vi "Analysis.Result Summaries, Generate Yield Per Day.vi"(9 "Type":enum16{"First Pass", "Last Pass", "All"}(ring), 11 "ResultSum":T1[](array[typedef])) -> (2 "Yield Per Date":string[][](table), 3 "Yield vs Date":cluster{timestamp[], dbl[]}(graph))   [LabVIEW 2024]
uses:
  Analysis.Result Summary.ctl
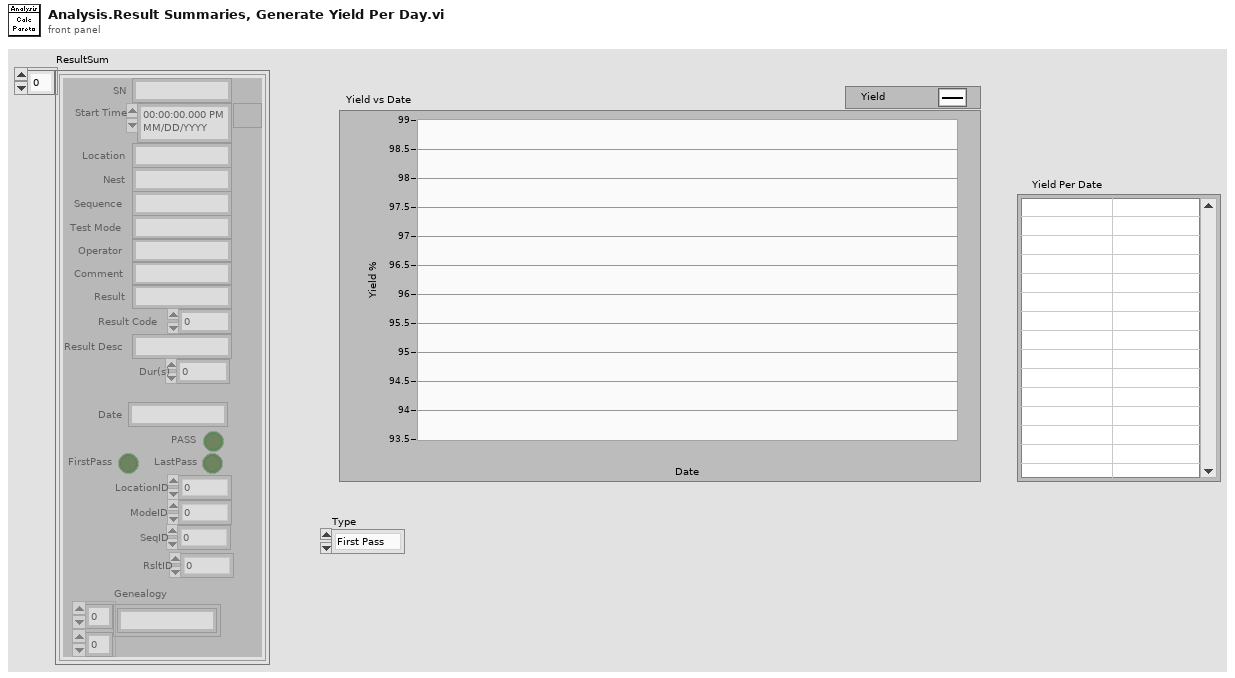
[diagram p1: front panel]
types:
  T1 = typedef "Analysis.Result Summary.ctl" = cluster{"SN":string, "Start Time":timestamp, "Location":string, "Nest":string, "Sequence":string, "Operator":string, "Test Mode":string, "Comment":string, "Result":string, "Result Code":i32, "Result Desc":string, "Date":string, "Dur(s)":dbl, "PASS":bool, "FirstPass":bool, "LastPass":bool, "LocationID":i32, "ModeID":i32, "SeqID":i32, "RsltID":i32, "Genealogy":string[][]}
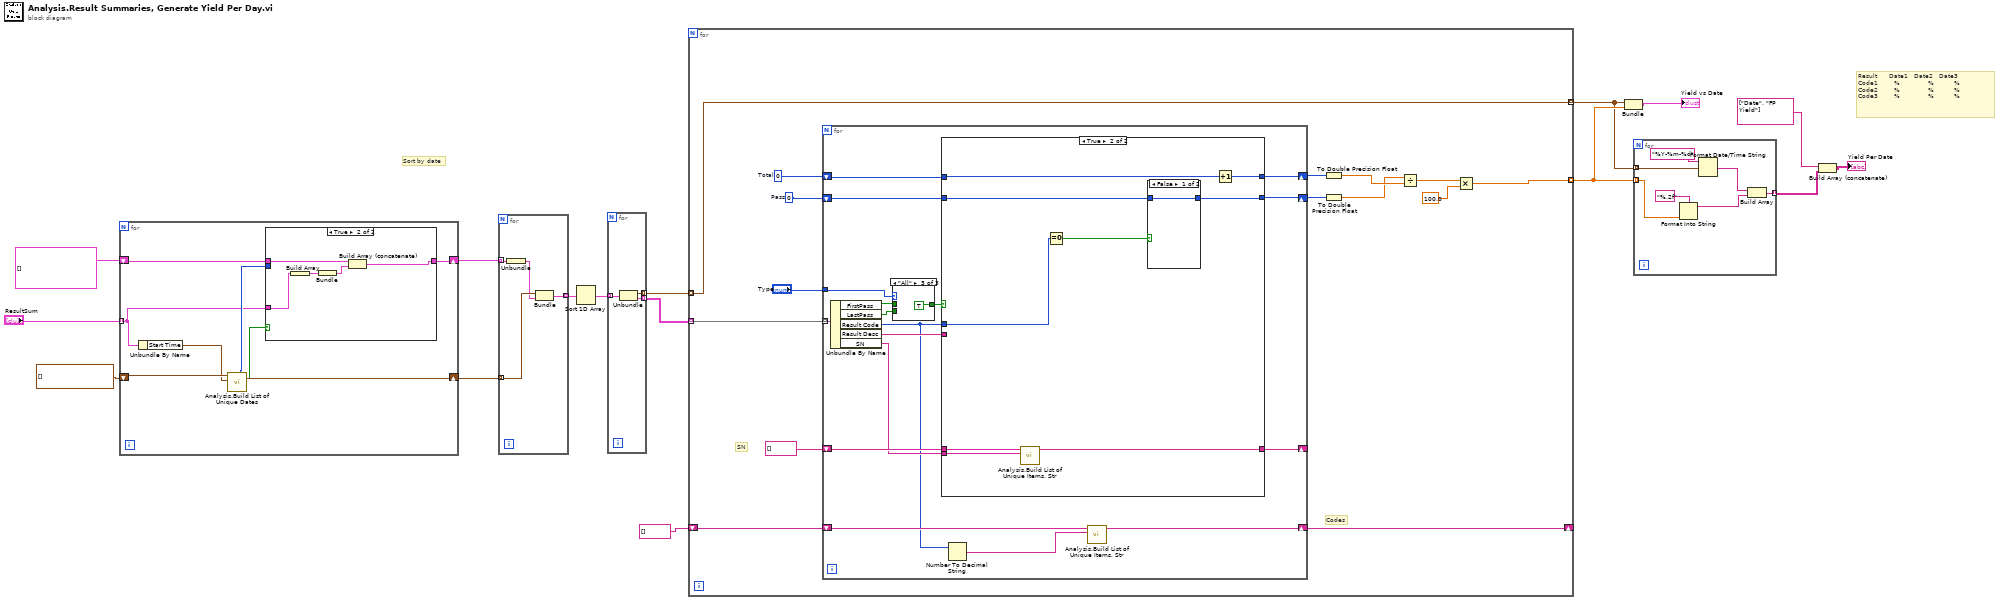
[diagram p0: block diagram]
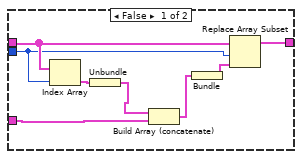
[diagram p2: hidden frame]
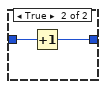
[diagram p6: hidden frame]
diagram:
  # "Sort by date"
  # "Result      Date1   Date2   Date3                 \nCode1        %              %          %\nCode2        %              %          %\nCode3        %              %          %"
  n1 = for {
    tunnel: "ResultSum" -> [w21] mode=indexing
    shift-right: [w23] -> w13
    shift-left: timestamp[] [] -> [w24]
    shift-right: [w18] -> w14
    shift-left: cluster{"ResultSum":T1[]}[] [] ("ResultSum") -> [w20]
    n2 = Unbundle By Name(w21) -> ("Start Time"=w17:timestamp)
    n3 = call "Analysis.Build List of Unique Dates.vi"("Date In"=w17, "Dates In"=w24) -> ("Added"=w19:bool, "Dates Out"=w23:timestamp[], "Index"=w22:i32)  [unwired: 7 in]
    n4 = case shown="True" w19 {
      tunnel: w22 -> [w31 _]
      tunnel: w21 -> [w30 w35]
      tunnel: w20 -> [w32 w37]
      tunnel: [w25 w36] -> w18
      frame False {
        n5 = Index Array(array=w32, index=w31) -> (element=w29:cluster{"ResultSum":T1[]})
        n6 = Unbundle(w29) -> ("ResultSum"=w28:T1[])
        n7 = Build Array (concatenate)(w28, w30) -> (w27:T1[])
        n8 = Bundle(w27) -> (w26:cluster{T1[]})  [unwired: 1 in]
        n9 = Replace Array Subset(array=w32, new element=w26, index=w31) -> (w25:cluster{"ResultSum":T1[]}[])
      }
      frame True {
        n10 = Build Array(w35) -> (w34:T1[])
        n11 = Bundle(w34) -> (w33:cluster{T1[]})  [unwired: 1 in]
        n12 = Build Array (concatenate)(w37, w33) -> (w36:cluster{"ResultSum":T1[]}[])
      }
    }
  }
  n13 = for {
    tunnel: w14 -> [w39] mode=indexing
    tunnel: w13 -> [w41] mode=indexing
    tunnel: [w40] -> w12 mode=indexing
    n14 = Unbundle(w39) -> ("ResultSum"=w38:T1[])
    n15 = Bundle("String"=w41, "ResultSum"=w38) -> (w40:cluster{"String":timestamp, "ResultSum":T1[]})  [unwired: 1 in]
  }
  n16 = Sort 1D Array(array=w12) -> (sorted array=w11:cluster{"String":timestamp, "ResultSum":T1[]}[])
  n17 = for {
    tunnel: w11 -> [w44] mode=indexing
    tunnel: [w43] -> w10 mode=indexing
    tunnel: [w42] -> w8 mode=indexing
    n18 = Unbundle(w44) -> ("String"=w42:timestamp, "ResultSum"=w43:T1[])
  }
  n19 = for {
    tunnel: w10 -> [w57] mode=indexing
    tunnel: w8 -> [w55] mode=indexing
    tunnel: [w55] -> w4 mode=indexing
    shift-right: [w53] -> _
    shift-left: string[] [] -> [w54]
    tunnel: [w45] -> w5 mode=indexing
    w52 = 0  # Pass
    w59 = 0  # Total
    # "Codes"
    # "SN"
    n20 = for {
      shift-right: [w75] -> w50
      shift-left: w52 -> [w76]
      tunnel: w57 -> [w72] mode=indexing
      shift-right: [w73] -> w51
      shift-left: w59 -> [w74]
      shift-right: [w68] -> _
      shift-left: string[] [] -> [w70]
      tunnel: "Type" -> [w67]
      shift-right: [w60] -> w53
      shift-left: w54 -> [w63]
      n21 = Unbundle By Name(w72) -> ("FirstPass"=w66:bool, "LastPass"=w65:bool, "Result Code"=w62:i32, "Result Desc"=w71:string, "SN"=w69:string)
      n22 = case shown="\"All\"" w67 {
        tunnel: w66 -> [w77 _ _]
        tunnel: w65 -> [_ w78 _]
        tunnel: [w77 w78 TRUE] -> w64
        frame "First Pass", Default {
        }
        frame "Last Pass" {
        }
        frame "All" {
        }
      }
      n23 = case shown="True" w64 {
        tunnel: w76 -> [w81 w84]
        tunnel: [w81 w83] -> w75
        tunnel: w74 -> [w82 w87]
        tunnel: [w82 w88] -> w73
        tunnel: w62 -> [_ w86]
        tunnel: w71 -> [_ _]
        tunnel: w70 -> [w80 w91]
        tunnel: w69 -> [_ w90]
        tunnel: [w80 w89] -> w68
        frame False {
        }
        frame True {
          n24 = call "Analysis.Build List of Unique Items, Str.vi"("Item In"=w90, "List In"=w91) -> ("List Out"=w89:string[])  [unwired: 7 in, 2 out]
          n25 = Equal To 0?(x=w86) -> (x = 0?=w85:bool)
          n26 = case shown="False" w85 {
            tunnel: w84 -> [w92 w94]
            tunnel: [w92 w93] -> w83
            frame False {
            }
            frame True {
              n27 = Increment(x=w94) -> (x+1=w93:i32)
            }
          }
          n28 = Increment(x=w87) -> (x+1=w88:i32)
        }
      }
      n29 = Number To Decimal String(number=w62) -> (decimal integer string=w61:string)  [unwired: 1 in]
      n30 = call "Analysis.Build List of Unique Items, Str.vi"("Item In"=w61, "List In"=w63) -> ("List Out"=w60:string[])  [unwired: 7 in, 2 out]
    }
    n31 = To Double Precision Float(number=w51) -> (double precision float=w49:dbl)
    n32 = To Double Precision Float(number=w50) -> (double precision float=w48:dbl)
    n33 = Divide(x=w48, y=w49) -> (x/y=w47:dbl)
    n34 = Multiply(x=w47, y=100.0) -> (x*y=w45:dbl)
  }
  n35 = Bundle(w4, w5) -> (→"Yield vs Date":cluster{timestamp[], dbl[]})  [unwired: 1 in]
  n36 = for {
    tunnel: w5 -> [w99] mode=indexing
    tunnel: w4 -> [w101] mode=indexing
    tunnel: [w95] -> w3 mode=indexing
    n37 = Format Into String(format string="%.2f", w99) -> (resulting string=w96:string)  [unwired: 2 in, 1 out]
    n38 = Format Date/Time String(time format string (%c)="%Y-%m-%d", seconds (now)=w101) -> (date/time string=w97:string)  [unwired: 1 in]
    n39 = Build Array(w97, w96) -> (w95:string[])
  }
  n40 = Build Array (concatenate)(string[] ["Date", "FP Yield"], w3) -> (→"Yield Per Date":string[][])
